vi "Process.vi"(8 "error in":errorcluster, 11 "Example Instrument UI":refnum<class "Instrument UI.Template.lvclass">) -> (0 "error out":errorcluster, 3 "Example Instrument UI out":refnum<class "Instrument UI.Template.lvclass">)   [LabVIEW 2019, in "Instrument UI.Template.lvclass"]
doc: "---------------------------------------------------------------\nJKI State Machine Objects™\nhttp://jki.net/state-machine-objects/\nCopyright (C) 2005-2015, JKI <info@jki.net>\nALL RIGHTS RESERVEDJKI State Machine Objects (SMO) 1.0.0.5\nJKI - JKI\nCopyright (c) 2016, JKI"
uses:
  Instrument UI.Template.lvclass
  C:/Program Files (x86)/National Instruments/LabVIEW 2019/vi.lib/JKI/JKI SMO/SMO/SMO.lvclass
  C:/Users/patrick/Documents/GitHub/Instrument-Framework/lvsrc/SMOs/Instrument UI/Instrument UI.lvclass
  C:/Program Files (x86)/National Instruments/LabVIEW 2019/vi.lib/JKI/JKI SMO/SMO.UI/SMO.UI.lvclass
  <vilib>/JKI/JKI SMO/SMO/Typedefs/Parent Call--Enum.ctl
  Instrument.Template/Typedefs/Instrument.Template.getAll--Cluster.ctl
  Instrument.Template/Instrument.Template.lvclass
  C:/Users/patrick/Documents/GitHub/Instrument-Framework/lvsrc/SMOs/Instrument/Instrument.lvclass
  Instrument UI.Template.UI--Cluster.ctl
  Instrument.Template/Typedefs/Instrument.Template.Configuration--Cluster.ctl
  SMOs/Configuration/Configuration.lvclass
  SMOs/Instrument UI/Instrument UI.lvclass/Instrument UI.ctl
  <vilib>/JKI/JKI SMO/SMO/SMO.lvclass/SMO.ctl
  SMOs/Instrument/Instrument.lvclass/Instrument.ctl
  614f1787-3484-4d72-b522-1f8c221dac07.vi
  064e3a37-d4cf-416d-9c97-81a00de9d50c.vi
  <vilib>/JKI/JKI SMO/SMO/Private/ReftoDVR--SMO.vi
  614f1787-3484-4d72-b522-1f8c221dac07.vi/599321bf-d042-4448-baa9-56506e4c2376.vi
  064e3a37-d4cf-416d-9c97-81a00de9d50c.vi/40046080-81aa-461f-9837-e8dd6f3bc5f2.vi
  614f1787-3484-4d72-b522-1f8c221dac07.vi/599321bf-d042-4448-baa9-56506e4c2376.vi/68c9d496-3a47-4762-a9a6-0350ec9b3b51.vi
  SMOs/Instrument/API/Send and Receive.vi
  064e3a37-d4cf-416d-9c97-81a00de9d50c.vi/40046080-81aa-461f-9837-e8dd6f3bc5f2.vi/33be0e9a-cf9b-4f8c-9dd9-f20244ed4396.vi
  614f1787-3484-4d72-b522-1f8c221dac07.vi/599321bf-d042-4448-baa9-56506e4c2376.vi/68c9d496-3a47-4762-a9a6-0350ec9b3b51.vi/238fe6a9-6a91-4c49-8d30-1c3fb86c5f8a.vi
  614f1787-3484-4d72-b522-1f8c221dac07.vi/599321bf-d042-4448-baa9-56506e4c2376.vi/68c9d496-3a47-4762-a9a6-0350ec9b3b51.vi/b5f16ff4-5c24-4e80-bad9-cd4679a5a0b8.vi
  064e3a37-d4cf-416d-9c97-81a00de9d50c.vi/40046080-81aa-461f-9837-e8dd6f3bc5f2.vi/33be0e9a-cf9b-4f8c-9dd9-f20244ed4396.vi/94746ab4-2c68-4577-8c39-bf3a51064162.vi
  064e3a37-d4cf-416d-9c97-81a00de9d50c.vi/40046080-81aa-461f-9837-e8dd6f3bc5f2.vi/33be0e9a-cf9b-4f8c-9dd9-f20244ed4396.vi/78597d36-8981-4427-a4ab-fc029080c8ad.vi
  SMOs/Instrument/API/Enum to String.vi
  SMOs/RemoteControl/API/Send and Receive.vi
  <vilib>/Utility/Data Type/Get Type Information.vi
  <vilib>/JDP Science/JSONtext/JSON text to Variant.vi
  SMOs/Instrument/Instrument.lvclass
  <vilib>/JDP Science/JSONtext/LVClass Serializer/JSONtext LVClass Serializer.lvclass
  SMOs/Instrument UI/Instrument UI.lvclass
  <vilib>/JKI/JKI SMO/SMO/SMO.lvclass
  <vilib>/JKI/JKI SMO/SMO.UI/SMO.UI.lvclass
panel:
  in  "Parameter 2":string
  out "Numeric":u32
  in  "Set Parameter":bool
  in  "Parameter":dbl
  in  "STOP":bool
  out "SMO string":string
  out "SMO Boolean":bool
  out "Logger SMO":dbl
  out "Levy 1":dbl
  # "#todo\nmake UI here. maybe include a nice picture of the hardware?"
  # "#todo\nadd buttons to do stuff (e.g., change a setting)\nButtons should trigger an event"
  # "#todo\nresize this box if you want your UI to be different size"
  # "SMO UI Template"
  # "For instructions on how to use the JKI State Machine Objects, examples and video tutorials, visit:\nhttp://jki.net/state-machine-objects/\n\nJKI State Machine Objects™\nhttp://jki.net/state-machine-objects/\nCopyright (C) 2005-2015, JKI <info@jki.net>\nALL RIGHTS RESERVED"
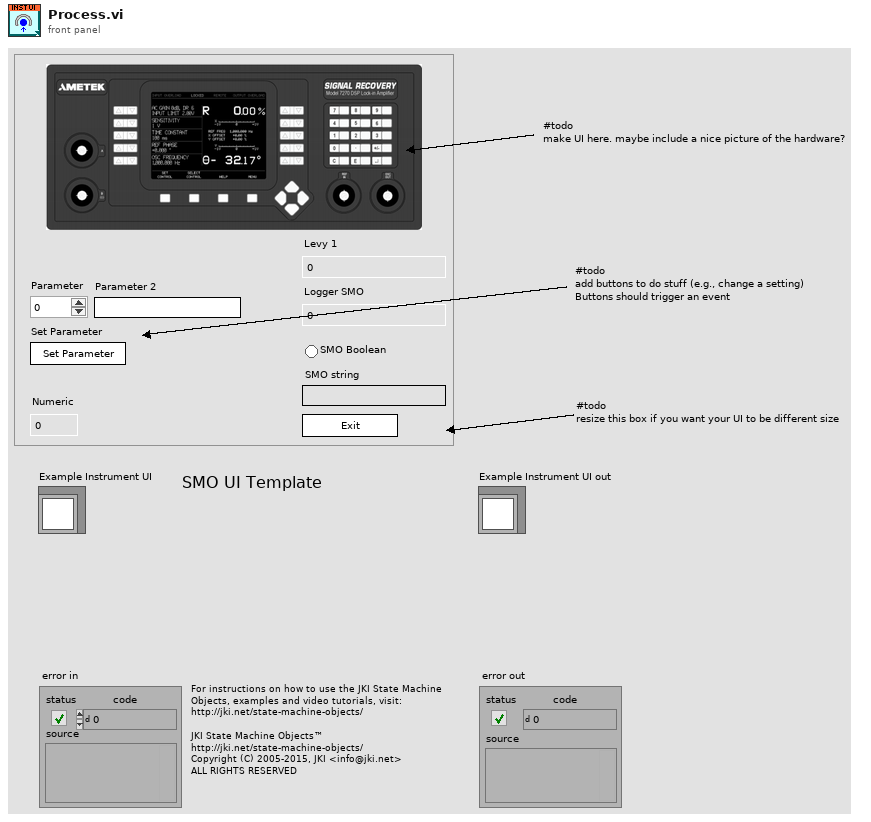
[diagram p1: front panel]
types:
  T1 = typedef "SMO.lvclass/Parent Call--Enum.ctl" = enum16{"Allows parent to run", "Does not request parent to run"}
  T2 = enum32{"invalid app kind", "Development System", "Run Time System", "Student Edition", "Embedded LabVIEW", "Evaluation", "Custom"}
  T3 = enum32{"Invalid", "Standard", "Closed", "Hidden", "Minimized", "Maximized"}
  T4 = typedef "Instrument.Template.lvclass/Instrument.Template.Configuration--Cluster.ctl" = cluster{"Example Setting 1":dbl, "Example Setting 2":dbl, "Example Setting 3":string}
  T5 = typedef "Instrument.Template.lvclass/Instrument.Template.getAll--Cluster.ctl" = cluster{"Levy 1":dbl, "Logger SMO":dbl, "SMO Boolean":bool, "SMO String":string}
  T6 = typedef "Instrument UI.Template.lvclass/Instrument UI.Template.UI--Cluster.ctl" = cluster{"Parameter":dbl, "Parameter 2":string}
  T7 = cluster{"Core":cluster{"Current VI Reference":refnum<vi>, "Close Panel on Exit?":bool, "error":errorcluster}, "Instrument UI":refnum<class "Instrument UI.Template.lvclass">, "Instrument":refnum<class "Instrument.Template.lvclass">, "Configuration":refnum<class "Configuration.lvclass">, "Config Cluster":T4, "getAll":T5, "UI Cluster":T6}
  T8 = cluster{"Current VI Reference":refnum<vi>, "Close Panel on Exit?":bool, "error":errorcluster}
  T9 = typedef "SMO.lvclass/Protected Events.ctl" = cluster{"StopProcesses":refnum<user-event>, "AbortProcesses":refnum<user-event>, "Config Changed":refnum<user-event>, "Dependency":refnum<user-event>}
  T10 = typedef "Instrument.lvclass/PublicEvents--Cluster.ctl" = cluster{"MessageFromProcess":refnum<user-event>}
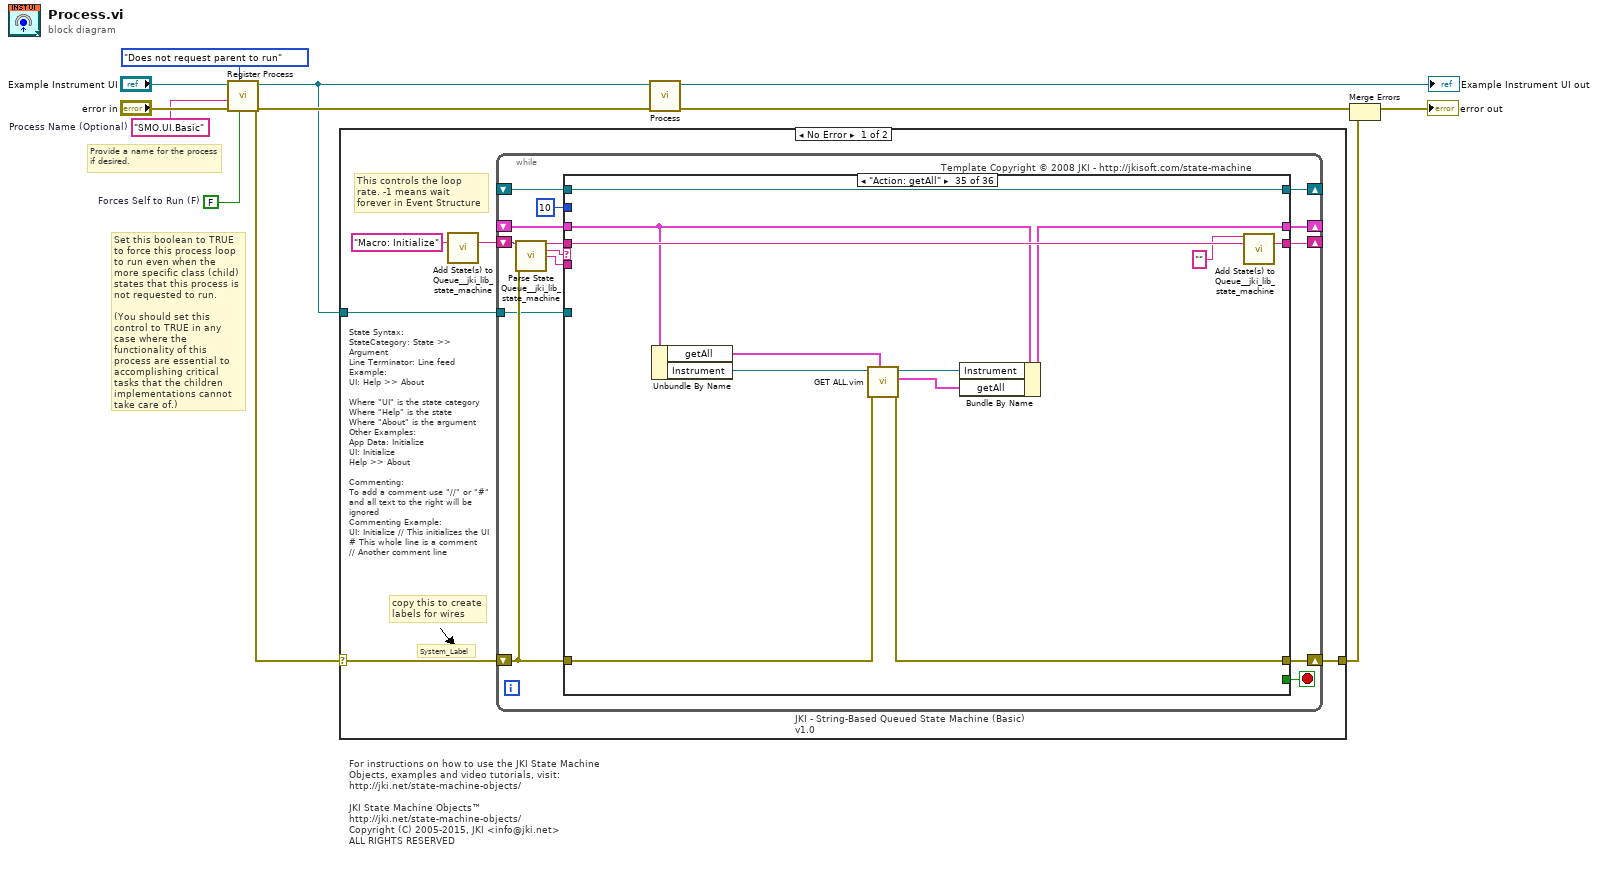
[diagram p0: block diagram]
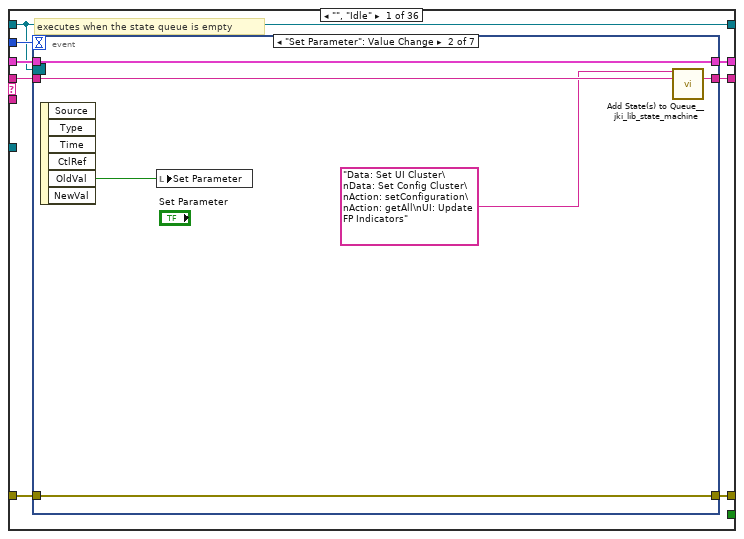
[diagram p2: hidden frame]
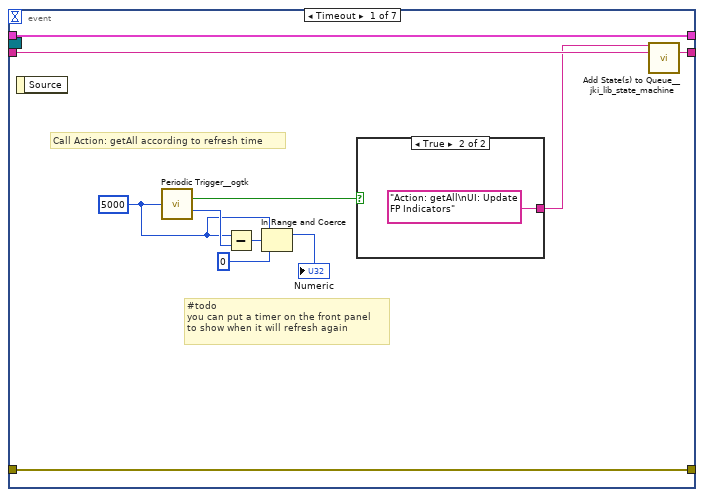
[diagram p3: hidden frame]
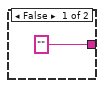
[diagram p4: hidden frame]
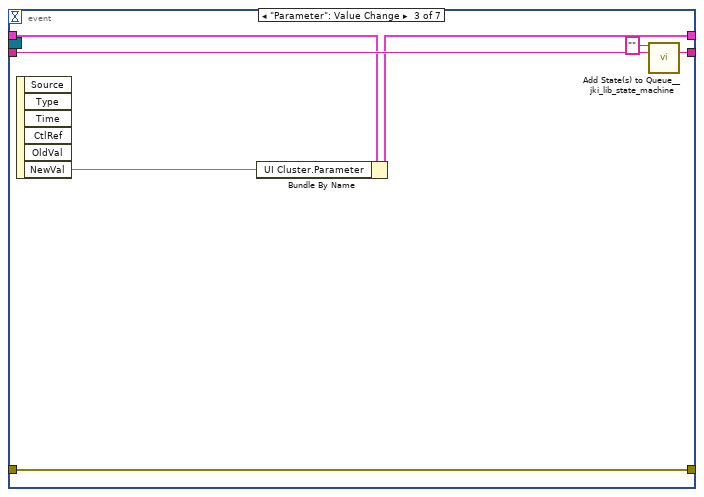
[diagram p5: hidden frame]
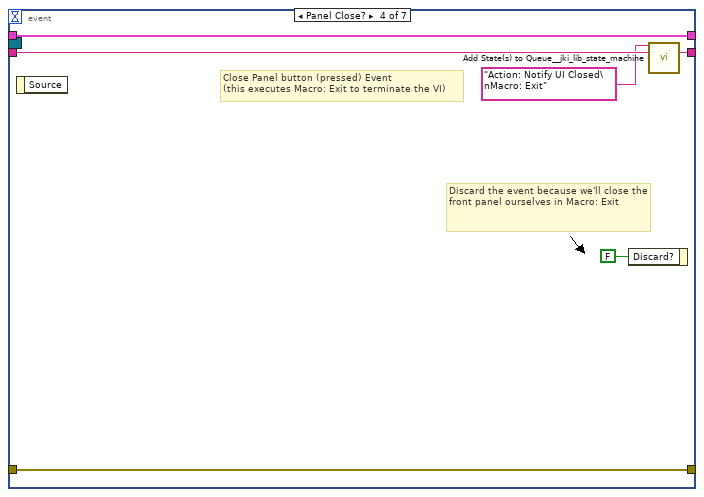
[diagram p6: hidden frame]
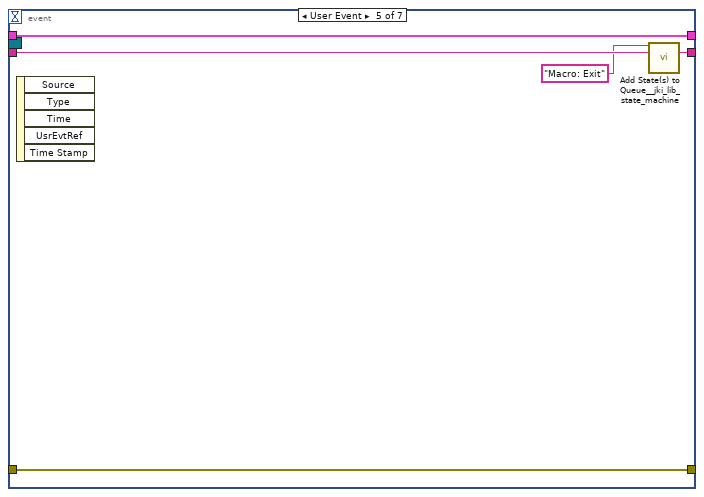
[diagram p7: hidden frame]
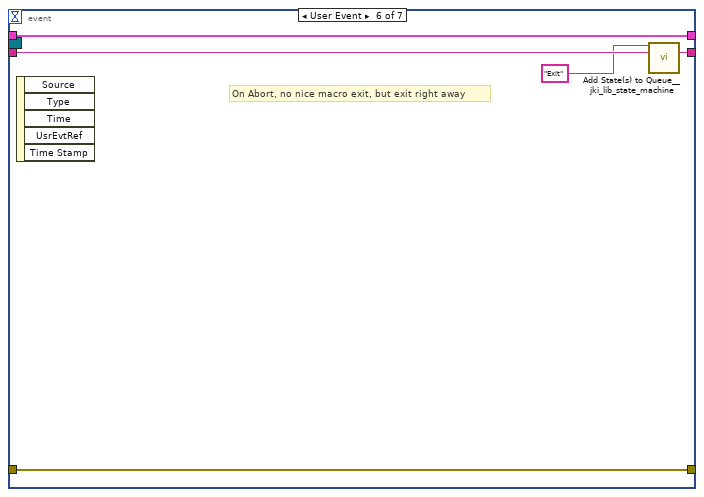
[diagram p8: hidden frame]
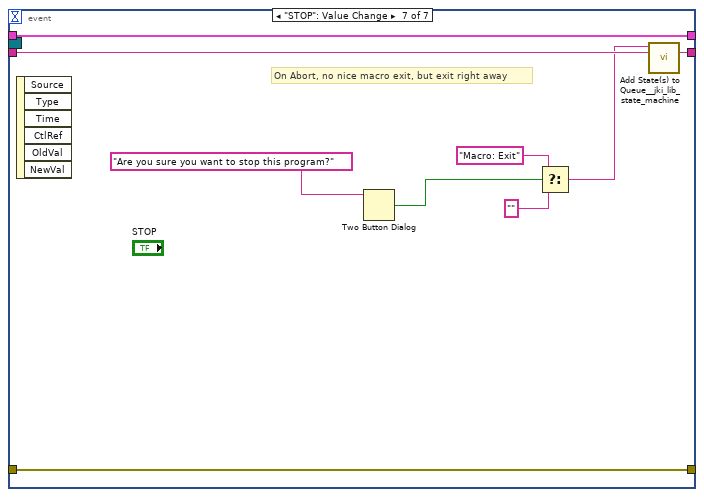
[diagram p9: hidden frame]
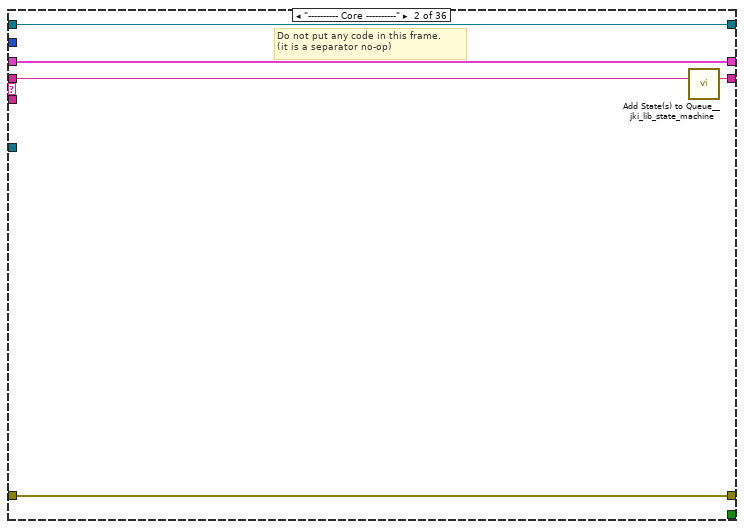
[diagram p10: hidden frame]
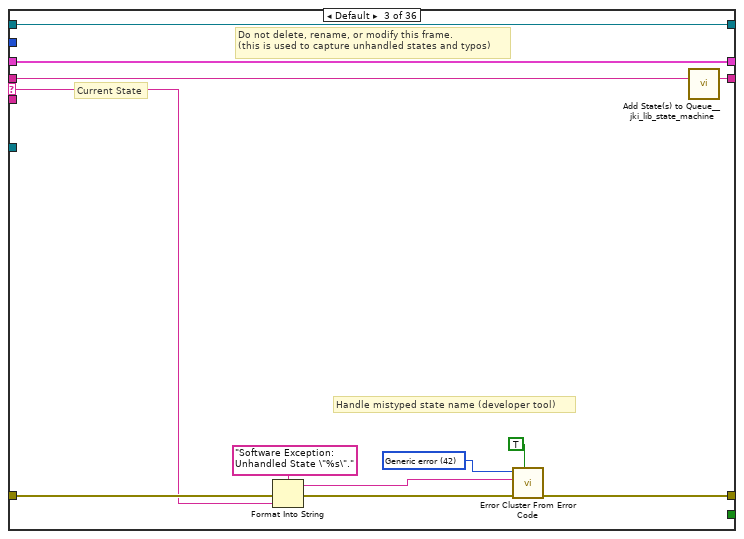
[diagram p11: hidden frame]
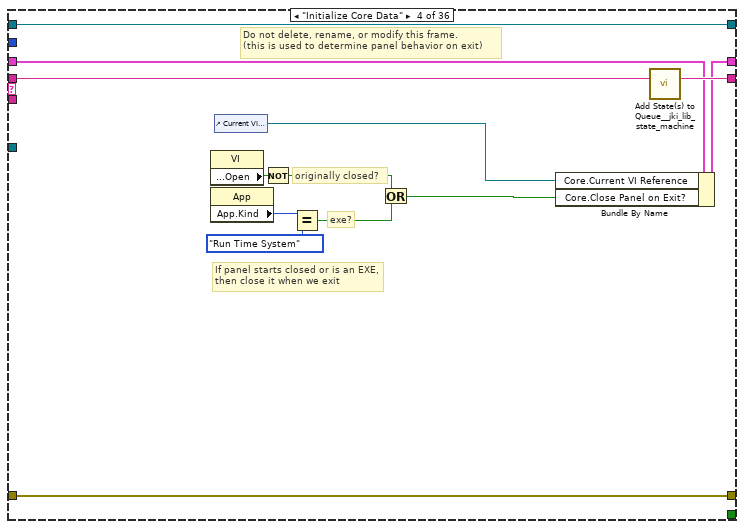
[diagram p12: hidden frame]
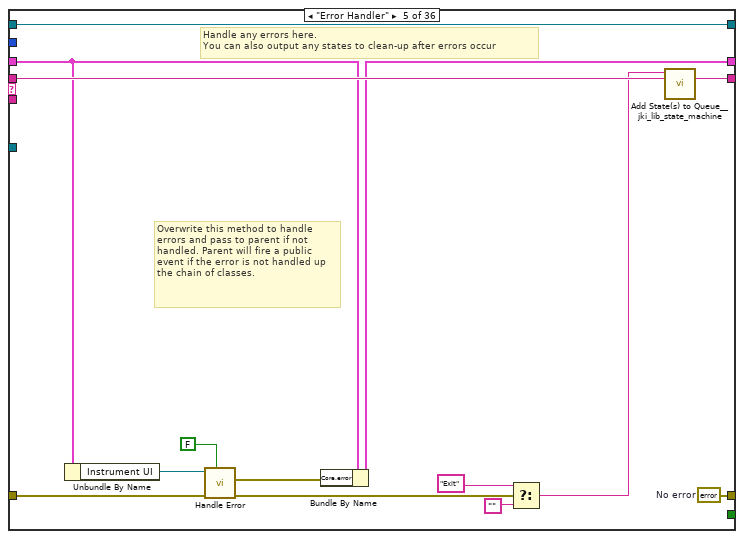
[diagram p13: hidden frame]
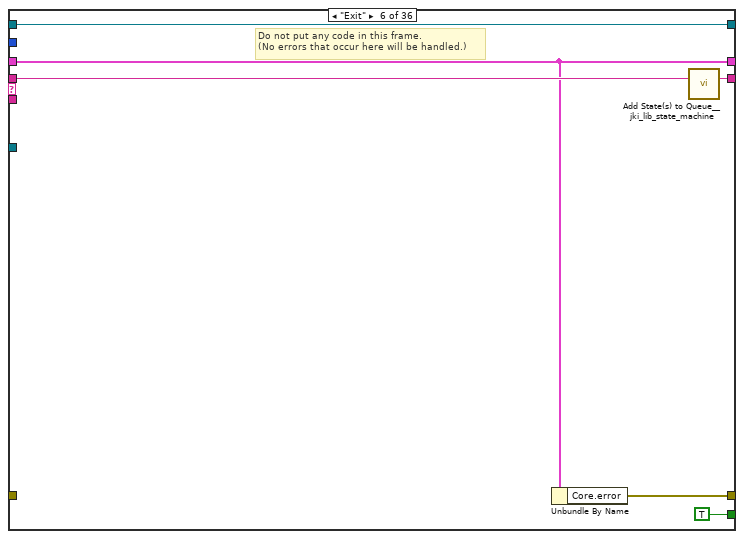
[diagram p14: hidden frame]
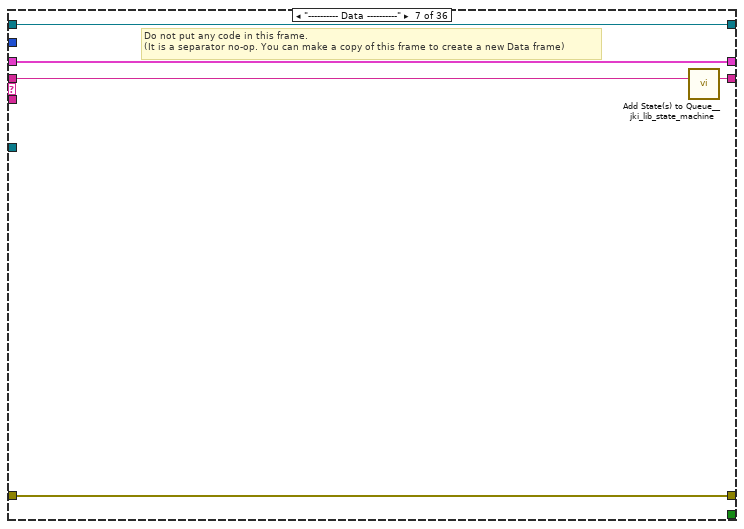
[diagram p15: hidden frame]
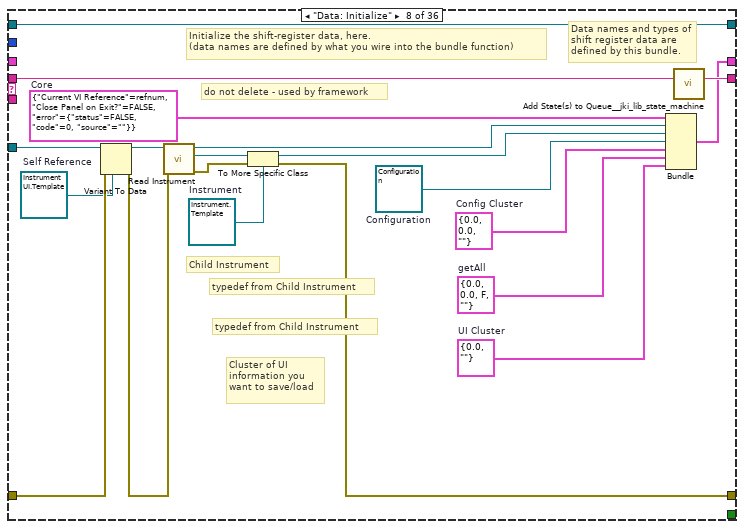
[diagram p16: hidden frame]
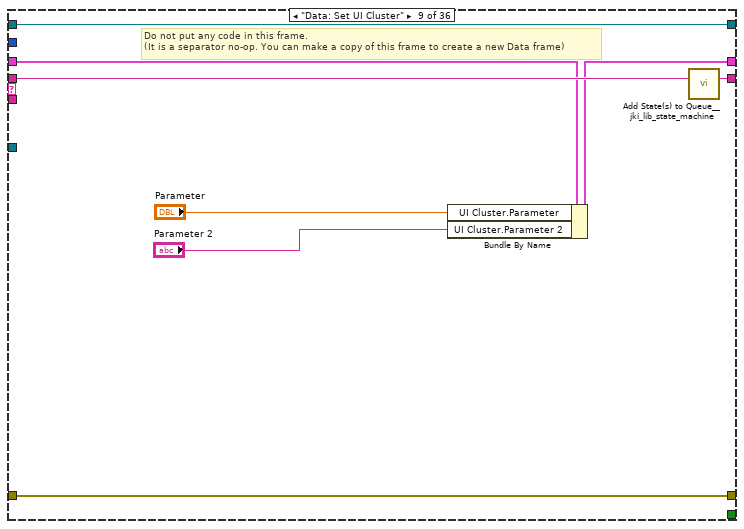
[diagram p17: hidden frame]
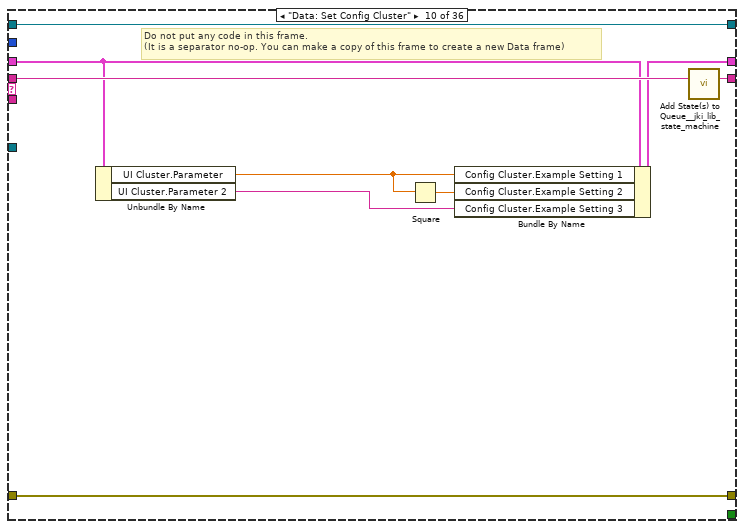
[diagram p18: hidden frame]
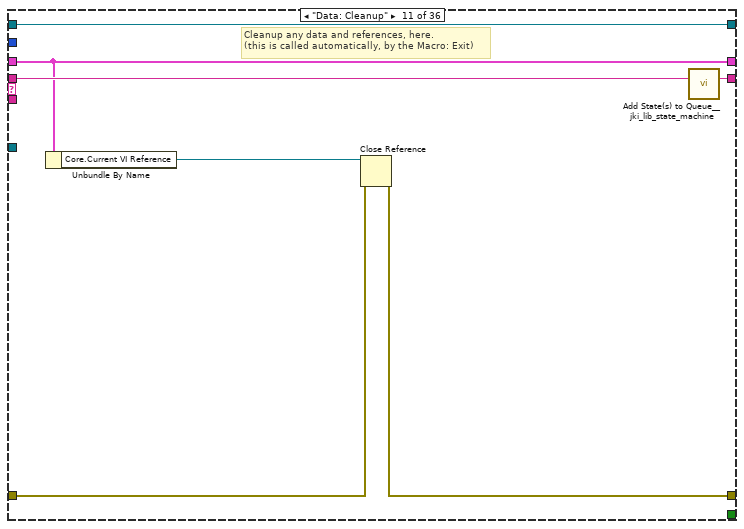
[diagram p19: hidden frame]
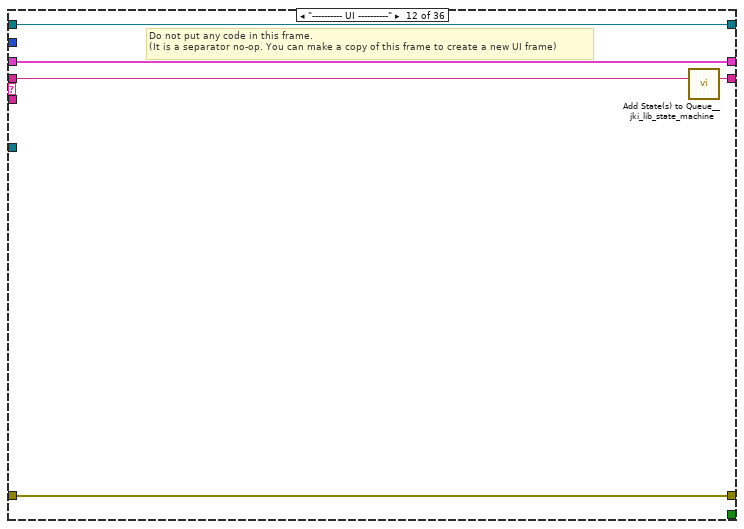
[diagram p20: hidden frame]
diagram:
  w2 = FALSE  # Forces Self to Run (F)
  w1 = "SMO.UI.Basic"  # Process Name (Optional)
  # "Provide a name for the process\nif desired."
  # "Set this boolean to TRUE to force this process loop to run even when the more specific class (child) states that this process is not requested to run.\n\n(You should set this control to TRUE in any case where the functionality of this process are essential to accomplishing critical tasks that the children implementations cannot take care of.)"
  # "For instructions on how to use the JKI State Machine Objects, examples and video tutorials, visit:\nhttp://jki.net/state-machine-objects/\n\nJKI State Machine Objects™\nhttp://jki.net/state-machine-objects/\nCopyright (C) 2005-2015, JKI <info@jki.net>\nALL RIGHTS RESERVED"
  n1 = call <vilib>:"Register Process.vi"("Forces Self to Run (F)"=w2, "Parent Call"=Parent_Call--Enum."Does not request parent to run", "error in (no error)"="error in", "Process Name (optional)"=w1, "SMO"="Example Instrument UI") -> ("error out"=w8:errorcluster, "SMO out"=w7:refnum<class "Instrument UI.Template.lvclass">)  [unwired: 5 in]
  n2 = case shown="No Error" w8 {
    selector: w8 -> [w13 w430]
    tunnel: w7 -> [w14 _]
    tunnel: [w12 w430] -> w4
    frame No Error {
      # "State Syntax:\nStateCategory: State >> Argument\nLine Terminator: Line feed\nExample:\nUI: Help >> About\n\nWhere \"UI\" is the state category\nWhere \"Help\" is the state\nWhere \"About\" is the argument\nOther Examples:\nApp Data: Initialize\nUI: Initialize\nHelp >> About\n\nCommenting:\nTo add a comment use \"//\" or \"#\" and all text to the right will be ignored\nCommenting Example:\nUI: Initialize // This initializes the UI\n# This whole line is a comment\n// Another comment line"
      # "copy this to create labels for wires"
      # "This controls the loop rate. -1 means wait forever in Event Structure"
      # "System_Label"
      n3 = call <vilib>:"Add State(s) to Queue__jki_lib_state_machine.vi"("State(s) in (\"\")"="Macro: Initialize") -> ("States Out"=w16:string)  [unwired: 14 in]
      n4 = while "JKI - String-Based Queued State Machine (Basic) v1.0" {
        shift-right: [w23] -> _
        shift-left: _ -> [w22]
        shift-right: [w26] -> w12
        shift-left: w13 -> [w20]
        shift-right: [w25] -> _
        shift-left: w16 -> [w27]
        tunnel: w14 -> [w19]
        shift-right: [w18] -> _
        shift-left: _ -> [w17]
        stop <- w24 stop-if-true
        # "Template Copyright © 2008 JKI - http://jkisoft.com/state-machine"
        n5 = call <vilib>:"Parse State Queue__jki_lib_state_machine.vi"("State Queue"=w27, "Error In (no error)"=w20) -> ("Remaining States"=w29:string, "Current State"=w30:string, "Arguments"=w28:string)  [unwired: 11 in]
        n6 = case shown="\"Action: getAll\"" w30 {
          selector: w30 -> [_ _ w96 _ _ _ _ _ _ _ _ _ _ _ _ _ _ _ _ _ _ _ _ _ _ _ _ _ _ _ _ _ _ _ _ _]
          tunnel: w29 -> [w38 w94 w100 w119 w133 w139 w144 w164 w172 w181 w188 w193 w200 w207 w217 w224 w240 w272 w281 w287 w293 w308 w313 w324 w331 w336 w349 w355 w360 w372 w380 w392 w399 w406 w418 w429]
          tunnel: w28 -> [_ _ _ _ _ _ _ _ _ _ _ _ _ _ _ w218 w234 _ _ _ _ _ _ _ _ _ _ _ _ _ _ _ _ _ _ _]
          tunnel: w22 -> [w36 w91 w98 w110 w122 w135 w141 _ w168 w177 w182 w190 w198 w203 w208 w222 w236 w269 w277 w284 w290 w295 w310 w321 w326 w333 w347 w353 w357 w363 w377 w383 w395 w400 w410 w421]
          tunnel: [w35 w92 w102 w116 w124 w134 w142 w146 w170 w179 w184 w191 w195 w205 w209 w219 w237 w270 w279 w285 w291 w306 w311 w315 w327 w334 w342 w350 w358 w367 w375 w384 w396 w401 w415 w426] -> w26
          tunnel: w20 -> [w34 w92 w101 w116 w129 _ w142 w161 w170 w179 w185 w191 w196 w205 w209 w220 w238 w270 w279 w285 w291 w306 w311 w316 w328 w334 w344 w351 w358 w365 w373 w385 w396 w402 w411 w422]
          tunnel: [w37 w93 w99 w118 w132 w138 w143 w163 w171 w180 w187 w192 w199 w206 w216 w223 w239 w271 w280 w286 w292 w307 w312 w323 w330 w335 w348 w354 w359 w371 w379 w391 w398 w405 w417 w428] -> w25
          tunnel: [_ _ _ _ _ TRUE _ _ _ _ _ _ _ _ _ _ _ _ _ _ _ _ _ _ _ _ _ _ _ _ _ _ _ _ _ _] -> w24
          tunnel: [w33 w91 w98 w117 w121 w135 w141 w162 w167 w176 w182 w190 w198 w203 w208 w222 w236 w269 w277 w284 w290 w295 w310 w321 w326 w333 w347 w353 w357 w369 w377 w381 w394 w400 w412 w423] -> w23
          tunnel: 10 ("Timeout") -> [w32 _ _ _ _ _ _ _ _ _ _ _ _ _ _ _ _ _ _ _ _ _ _ _ _ _ _ _ _ _ _ _ _ _ _ _]
          tunnel: w19 -> [_ _ _ _ _ _ _ w159 _ _ _ _ _ _ _ _ _ _ _ _ _ _ _ _ _ _ _ _ _ _ _ _ _ _ _ _]
          tunnel: [w31 w90 w95 w107 w131 w136 w140 w158 w169 w178 w183 w189 w197 w204 w215 w221 w233 w268 w278 w283 w289 w300 w309 w322 w329 w332 w346 w352 w356 w370 w378 w390 w397 w404 w416 w427] -> w18
          tunnel: w17 -> [w31 w90 w95 w107 w131 w136 w140 w158 w169 w178 w183 w189 w197 w204 w215 w221 w233 w268 w278 w283 w289 w300 w309 w322 w329 w332 _ w352 w356 w370 w378 w390 w397 w404 w416 w427]
          frame "", "Idle" {
            # "executes when the state queue is empty"
            n7 = event shown="[1] \"Set Parameter\": Value Change" {
              selector: w31 -> [_ _ _ _ _ _ _]
              dyn-events: _ -> [_ _ _ _ _ _ _]
              timeout: w32 -> [_ _ _ _ _ _ _]
              tunnel: w38 -> [w49 w57 w64 w70 w75 w80 w89]
              tunnel: [w48 w56 w63 w69 w74 w79 w88] -> w37
              tunnel: w36 -> [w46 w54 w60 w66 w72 w77 w86]
              tunnel: [w47 w55 w62 w65 w73 w78 w87] -> w35
              tunnel: w34 -> [w47 w55 w62 w65 w73 w78 w87]
              tunnel: [w46 w54 w59 w66 w72 w77 w86] -> w33
              event Timeout {
                w40 = u32 5000 ("time (ms)")
                # "#todo\nyou can put a timer on the front panel\nto show when it will refresh again"
                # "Call Action: getAll according to refresh time"
                n8 = event-data() -> ()  [unwired: 1 in, 1 out]
                n9 = call <userlib>:"Periodic Trigger__ogtk.vi"("time (ms)"=w40) -> ("Triggered"=w44:bool, "timer value"=w43:u32)  [unwired: 12 in, 1 out]
                n10 = Subtract(x=w40, y=w43) -> (x-y=w42:u32)
                n11 = In Range and Coerce(upper limit=w40, x=w42, lower limit=u32 0) -> (coerced(x)=→"Numeric":u32)  [unwired: 1 out]
                n12 = case shown="True" w44 {
                  tunnel: ["" ("State(s) in Front (\"\")") "Action: getAll\nUI: Update FP Indicators" ("State(s) in Front (\"\")")] -> w45
                  frame False {
                  }
                  frame True {
                  }
                }
                n13 = call <vilib>:"Add State(s) to Queue__jki_lib_state_machine.vi"("State(s) in Front (\"\")"=w45, "State(s) in (\"\")"=w49) -> ("States Out"=w48:string)  [unwired: 13 in]
              }
              event "Set Parameter": Value Change {
                n14 = event-data() -> ("OldVal"=w53:bool)  [unwired: 1 in, 5 out]
                n15 = local write "Set Parameter"(w53) -> ()
                n16 = call <vilib>:"Add State(s) to Queue__jki_lib_state_machine.vi"("State(s) in Front (\"\")"="Data: Set UI Cluster\nData: Set Config Cluster\nAction: setConfiguration\nAction: getAll\nUI: Update FP Indicators" ("State(s) in Front (\"\")"), "State(s) in (\"\")"=w57) -> ("States Out"=w56:string)  [unwired: 13 in]
              }
              event "Parameter": Value Change {
                n17 = event-data() -> ("NewVal"=w61:dbl)  [unwired: 1 in, 5 out]
                n18 = Bundle By Name(cluster=w60, "UI Cluster.Parameter"=w61) -> (w59:T7)
                n19 = call <vilib>:"Add State(s) to Queue__jki_lib_state_machine.vi"("State(s) in Front (\"\")"="" ("State(s) in Front (\"\")"), "State(s) in (\"\")"=w64) -> ("States Out"=w63:string)  [unwired: 13 in]
              }
              event Panel Close? {
                # "Discard the event because we'll close the front panel ourselves in Macro: Exit"
                # "Close Panel button (pressed) Event\n(this executes Macro: Exit to terminate the VI)"
                n20 = event-data() -> ()  [unwired: 1 in, 1 out]
                n21 = event-data("Discard?"=FALSE) -> ()  [unwired: 1 in, 1 out]
                n22 = call <vilib>:"Add State(s) to Queue__jki_lib_state_machine.vi"("State(s) in Front (\"\")"="Action: Notify UI Closed\nMacro: Exit", "State(s) in (\"\")"=w70) -> ("States Out"=w69:string)  [unwired: 13 in]
              }
              event User Event {
                n23 = event-data() -> ()  [unwired: 1 in, 5 out]
                n24 = call <vilib>:"Add State(s) to Queue__jki_lib_state_machine.vi"("State(s) in Front (\"\")"="Macro: Exit", "State(s) in (\"\")"=w75) -> ("States Out"=w74:string)  [unwired: 13 in]
              }
              event User Event {
                # "On Abort, no nice macro exit, but exit right away"
                n25 = event-data() -> ()  [unwired: 1 in, 5 out]
                n26 = call <vilib>:"Add State(s) to Queue__jki_lib_state_machine.vi"("State(s) in Front (\"\")"="Exit", "State(s) in (\"\")"=w80) -> ("States Out"=w79:string)  [unwired: 13 in]
              }
              event "STOP": Value Change {
                # "On Abort, no nice macro exit, but exit right away"
                n27 = event-data() -> ()  [unwired: 1 in, 6 out]
                n28 = Two Button Dialog(message="Are you sure you want to stop this program?") -> (T button?=w85:bool)  [unwired: 2 in]
                n29 = Select(t="Macro: Exit", s=w85, f="") -> (s? t:f=w81:string)
                n30 = call <vilib>:"Add State(s) to Queue__jki_lib_state_machine.vi"("State(s) in Front (\"\")"=w81, "State(s) in (\"\")"=w89) -> ("States Out"=w88:string)  [unwired: 13 in]
              }
            }
          }
          frame "---------- Core ----------" {
            # "Do not put any code in this frame.\n(it is a separator no-op)"
            n31 = call <vilib>:"Add State(s) to Queue__jki_lib_state_machine.vi"("State(s) in (\"\")"=w94) -> ("States Out"=w93:string)  [unwired: 14 in]
          }
          frame Default {
            w105 = 42 items=["No error", "Argument error", "Memory is full", "Out of zone", "End of file", "File already open", "Generic file I/O error", "File not found", "File permission error", "Disk is full", "Duplicate path", "Too many files open", "System feature not enabled", "Resource file not found", "Cannot add resource", "Resource not found", "Image not found", "Image memory error", "Pen does not exist", "Config type invalid", "Config token not found", "Config parse error", "Config memory error", "Bad external code format", "Bad external code offset", "External code not present", "Null window", "Destroy window error", "Null menu", "Print aborted", "Bad print record", "Print driver error", "Windows error during printing", "Memory error during printing", "Print dialog error", "Generic print error", "Invalid device refnum", "Device not found", "Device parameter error", "Device unit error", "Cannot open device", "Device call aborted", "Generic error", "Cancelled by user", "Object ID too low", "Object ID too high", "Object not in heap", "Unknown heap", "Unknown object (invalid DefProc)", "Unknown object (DefProc not in table)", "Message out of range", "Invalid (null) method", "Unknown message", "Manager call not supported", "Bad address", "Network operation in progress", "Network operation timed out", "Connection is busy", "Network attribute not supported", "Network error", "Address in use", "System out of memory", "Connection aborted", "Connection refused", "Not connected", "Already connected", "Connection closed", "Initialization error (interapplication manager)", "Bad occurrence", "Wait on unbound occurrence handler", "Occurrence queue overflow", "Datalog type conflict", "Unused", "Unrecognized type (interapplication manager)", "Memory corrupt", "Failed to make temporary DLL", "Old CIN version", "Drag socket not found", "Failed to load drop-object", "Failed to register OLE object", "Failed to release OLE object", "Format specifier type mismatch", "Unknown format specifier", "Too few format specifiers", "Too many format specifiers", "Scan failed", "Newer CIN version", "Error converting to variant", "Runtime menu error", "Password tampered", "Variant attribute not found", "Incompatible variant data type", "Event data is not available", "Event Store is not present", "Occurrence is not found", "Event Queue is not created", "Event info is not available", "Refnum passed is NULL", "Error retrieving Class GUID", "Error retrieving CoClass GUID", "Error retrieving TypeLib GUID.", "Bad built application magic bytes.", "Specific driver is different from the specific driver associated with the Logical Name.", "There is no session opened to the class driver.", "Max Error", "MAX - Error with config objects", "MAX - Error loading configuration", "MAX - Group not supported"]
            # "Current State"
            # "Do not delete, rename, or modify this frame.\n(this is used to capture unhandled states and typos)"
            # "Handle mistyped state name (developer tool)"
            n32 = Format Into String(format string="Software Exception: Unhandled State \"%s\"." ("message"), error in=w101, w96) -> (resulting string=w104:string, error out=w103:errorcluster)  [unwired: 1 in]
            n33 = call <vilib>:"Error Cluster From Error Code.vi"("show call chain? (False)"=TRUE, "error in (no error)"=w103, "error message (\"\")"=w104, "error code (0)"=w105) -> ("error out"=w102:errorcluster)  [unwired: 5 in]
            n34 = call <vilib>:"Add State(s) to Queue__jki_lib_state_machine.vi"("State(s) in (\"\")"=w100) -> ("States Out"=w99:string)  [unwired: 14 in]
          }
          frame "Initialize Core Data" {
            # "Do not delete, rename, or modify this frame.\n(this is used to determine panel behavior on exit)"
            # "originally closed?"
            # "exe?"
            # "If panel starts closed or is an EXE, then close it when we exit"
            n35 = property class="VI"() -> ("Front Panel.Open"=w115:bool)  [unwired: 2 in, 2 out]
            n36 = property class="App"() -> ("App.Kind"=w114:T2)  [unwired: 2 in, 2 out]
            n37 = control-ref of="Current VI Reference"() -> (w108:refnum<vi>)
            n38 = Not(x=w115) -> (.not. x?=w112:bool)
            n39 = Equal?(x=w114, y=T2."Run Time System" ("Application:Kind")) -> (x = y?=w111:bool)
            n40 = Or(x=w112, y=w111) -> (x .or. y?=w109:bool)
            n41 = Bundle By Name(cluster=w110, "Core.Current VI Reference"=w108, "Core.Close Panel on Exit?"=w109) -> (w117:T7)
            n42 = call <vilib>:"Add State(s) to Queue__jki_lib_state_machine.vi"("State(s) in (\"\")"=w119) -> ("States Out"=w118:string)  [unwired: 14 in]
          }
          frame "Error Handler" {
            w124 = errorcluster {"status"=FALSE, "code"=0, "source"=""}  # No error
            # "Overwrite this method to handle errors and pass to parent if not handled. Parent will fire a public event if the error is not handled up the chain of classes."
            # "Handle any errors here.\nYou can also output any states to clean-up after errors occur"
            n43 = Unbundle By Name(w122) -> ("Instrument UI"=w130:refnum<class "Instrument UI.Template.lvclass">)
            n44 = call-dynamic "Handle Error.vi"("Stop on Unhandled Error (T)"=FALSE, "error in"=w129, "SMO"=w130) -> ("handling error"=w125:errorcluster, "Unhandled error"=w123:errorcluster)  [unwired: 6 in, 1 out]
            n45 = Bundle By Name(cluster=w122, "Core.error"=w123) -> (w121:T7)
            n46 = Select(t="Exit", s=w125, f="") -> (s? t:f=w126:string)
            n47 = call <vilib>:"Add State(s) to Queue__jki_lib_state_machine.vi"("State(s) in Front (\"\")"=w126, "State(s) in (\"\")"=w133) -> ("States Out"=w132:string)  [unwired: 13 in]
          }
          frame "Exit" {
            # "Do not put any code in this frame.\n(No errors that occur here will be handled.)"
            n48 = Unbundle By Name(w135) -> ("Core.error"=w134:errorcluster)
            n49 = call <vilib>:"Add State(s) to Queue__jki_lib_state_machine.vi"("State(s) in (\"\")"=w139) -> ("States Out"=w138:string)  [unwired: 14 in]
          }
          frame "---------- Data ----------" {
            # "Do not put any code in this frame.\n(It is a separator no-op. You can make a copy of this frame to create a new Data frame)"
            n50 = call <vilib>:"Add State(s) to Queue__jki_lib_state_machine.vi"("State(s) in (\"\")"=w144) -> ("States Out"=w143:string)  [unwired: 14 in]
          }
          frame "Data: Initialize" {
            w145 = refnum<class "Configuration.lvclass"> refnum  # Configuration
            w148 = T4 {"Example Setting 1"=0.0, "Example Setting 2"=0.0, "Example Setting 3"=""}  # Config Cluster
            w150 = T6 {"Parameter"=0.0, "Parameter 2"=""}  # UI Cluster
            w152 = refnum<class "Instrument.Template.lvclass"> refnum  # Instrument
            w156 = T5 {"Levy 1"=0.0, "Logger SMO"=0.0, "SMO Boolean"=FALSE, "SMO String"=""}  # getAll
            w157 = T8 {"Current VI Reference"=refnum, "Close Panel on Exit?"=FALSE, "error"={"status"=FALSE, "code"=0, "source"=""}}  # Core
            w160 = refnum<class "Instrument UI.Template.lvclass"> refnum  # Self Reference
            # "typedef from Child Instrument"
            # "Cluster of UI\ninformation you\nwant to save/load"
            # "Child Instrument"
            # "typedef from Child Instrument"
            # "do not delete - used by framework"
            # "Data names and types of shift register data are defined by this bundle."
            # "Initialize the shift-register data, here.\n(data names are defined by what you wire into the bundle function)"
            n51 = Variant To Data(error in=w161, type=w160, Variant=w159) -> (data=w154:refnum<class "Instrument UI.Template.lvclass">, error out=w155:errorcluster)
            n52 = call "Read Instrument.vi"("error in (no error)"=w155, "Instrument UI in"=w154) -> ("error out"=w149:errorcluster, "Instrument"=w151:refnum<class "Instrument.lvclass">, "Instrument UI"=w153:refnum<class "Instrument UI.Template.lvclass">)  [unwired: 7 in]
            n53 = To More Specific Class(target class=w152, reference=w151, error in=w149) -> (specific class reference=w147:refnum<class "Instrument.Template.lvclass">, error out=w146:errorcluster)
            n54 = Bundle("Core"=w157, "Instrument UI"=w153, "Instrument"=w147, "Configuration"=w145, "Config Cluster"=w148, "getAll"=w156, "UI Cluster"=w150) -> (w162:T7)  [unwired: 1 in]
            n55 = call <vilib>:"Add State(s) to Queue__jki_lib_state_machine.vi"("State(s) in (\"\")"=w164) -> ("States Out"=w163:string)  [unwired: 14 in]
          }
          frame "Data: Set UI Cluster" {
            # "Do not put any code in this frame.\n(It is a separator no-op. You can make a copy of this frame to create a new Data frame)"
            n56 = Bundle By Name(cluster=w168, "UI Cluster.Parameter"="Parameter", "UI Cluster.Parameter 2"="Parameter 2") -> (w167:T7)
            n57 = call <vilib>:"Add State(s) to Queue__jki_lib_state_machine.vi"("State(s) in (\"\")"=w172) -> ("States Out"=w171:string)  [unwired: 14 in]
          }
          frame "Data: Set Config Cluster" {
            # "Do not put any code in this frame.\n(It is a separator no-op. You can make a copy of this frame to create a new Data frame)"
            n58 = Unbundle By Name(w177) -> ("UI Cluster.Parameter"=w174:dbl, "UI Cluster.Parameter 2"=w175:string)
            n59 = Square(x=w174) -> (x^2=w173:dbl)
            n60 = Bundle By Name(cluster=w177, "Config Cluster.Example Setting 1"=w174, "Config Cluster.Example Setting 2"=w173, "Config Cluster.Example Setting 3"=w175) -> (w176:T7)
            n61 = call <vilib>:"Add State(s) to Queue__jki_lib_state_machine.vi"("State(s) in (\"\")"=w181) -> ("States Out"=w180:string)  [unwired: 14 in]
          }
          frame "Data: Cleanup" {
            # "Cleanup any data and references, here.\n(this is called automatically, by the Macro: Exit)"
            n62 = Unbundle By Name(w182) -> ("Core.Current VI Reference"=w186:refnum<vi>)
            n63 = Close Reference(reference=w186, error in (no error)=w185) -> (error out=w184:errorcluster)
            n64 = call <vilib>:"Add State(s) to Queue__jki_lib_state_machine.vi"("State(s) in (\"\")"=w188) -> ("States Out"=w187:string)  [unwired: 14 in]
          }
          frame "---------- UI ----------" {
            # "Do not put any code in this frame.\n(It is a separator no-op. You can make a copy of this frame to create a new UI frame)"
            n65 = call <vilib>:"Add State(s) to Queue__jki_lib_state_machine.vi"("State(s) in (\"\")"=w193) -> ("States Out"=w192:string)  [unwired: 14 in]
          }
          frame "UI: Initialize" {
            # "size window to decoration box on front panel"
            # "Initialize the User Interface, here.\n(this is called automatically, by the Macro: Init)"
            n66 = invoke on="STOP" class="Bool (strict)" method="Reinit To Default"() -> ()  [unwired: 3 in, 3 out]
            n67 = call <userlib>:"Fit VI window to Largest Dec__ogtk.vi"("error in (no error)"=w196, "border spacing (2 px)"=0) -> ("error out"=w195:errorcluster)  [unwired: 4 in, 1 out]
            n68 = call <vilib>:"Add State(s) to Queue__jki_lib_state_machine.vi"("State(s) in (\"\")"=w200) -> ("States Out"=w199:string)  [unwired: 14 in]
          }
          frame "UI: Update FP Controls" {
            # "Do not put any code in this frame.\n(It is a separator no-op. You can make a copy of this frame to create a new UI frame)"
            n69 = Unbundle By Name(w203) -> ("UI Cluster.Parameter"=w201:dbl, "UI Cluster.Parameter 2"=w202:string)
            n70 = local write "Parameter 2"(w202) -> ()
            n71 = local write "Parameter"(w201) -> ()
            n72 = call <vilib>:"Add State(s) to Queue__jki_lib_state_machine.vi"("State(s) in (\"\")"=w207) -> ("States Out"=w206:string)  [unwired: 14 in]
          }
          frame "UI: Update FP Indicators" {
            # "do this way to have nicer UI or only display what you want"
            n73 = Unbundle By Name(w208) -> ("getAll"=w210:T5)
            n74 = Unbundle By Name(w210) -> ("Levy 1"=→"Levy 1":dbl, "Logger SMO"=→"Logger SMO":dbl, "SMO Boolean"=→"SMO Boolean":bool, "SMO String"=→"SMO string":string)
            n75 = call <vilib>:"Add State(s) to Queue__jki_lib_state_machine.vi"("State(s) in (\"\")"=w217) -> ("States Out"=w216:string)  [unwired: 14 in]
          }
          frame "UI: Cursor Set" {
            # "Argument"
            # "Initialize the User Interface, here.\n(this is called automatically, by the Macro: Init)"
            n76 = disable-structure shown="Default" {
              disable-tunnel: w220 -> [w225 w228]
              disable-tunnel: [w225 w227] -> w219
              disable-tunnel: w218 -> [_ w226]
              frame condition #0 {
              }
              frame condition #1 (active) {
                n77 = case shown="\"Busy\"" w226 {
                  tunnel: w228 -> [w230 w232]
                  tunnel: [w229 w231] -> w227
                  frame "Idle", Default {
                    n78 = call <vilib>:"Unset Busy.vi"("error in (no error)"=w230) -> ("error out"=w229:errorcluster)  [unwired: 10 in]
                  }
                  frame "Busy" {
                    n79 = call <vilib>:"Set Busy.vi"("error in (no error)"=w232) -> ("error out"=w231:errorcluster)  [unwired: 9 in, 1 out]
                  }
                }
              }
            }
            n80 = call <vilib>:"Add State(s) to Queue__jki_lib_state_machine.vi"("State(s) in (\"\")"=w224) -> ("States Out"=w223:string)  [unwired: 14 in]
          }
          frame "UI: Front Panel State" {
            # "Argument"
            # "Set Front Panel Open or Closed\n(Usage: \"UI: Front Panel State >> Open|Close\")"
            n81 = Unbundle By Name(w236) -> ("Core.Current VI Reference"=w235:refnum<vi>)
            n82 = disable-structure shown="Default" {
              disable-tunnel: w238 -> [w244 w267]
              disable-tunnel: [w243 w267] -> w237
              disable-tunnel: w235 -> [w242 _]
              disable-tunnel: w234 -> [w241 _]
              frame condition #0 (active) {
                n83 = case shown="\"Close\"" w241 {
                  tunnel: w244 -> [w248 w261]
                  tunnel: [w250 w262] -> w243
                  tunnel: w242 -> [w249 w259]
                  frame "Open", Default {
                    n84 = property class="VI"(reference=w249, error in=w248) -> (reference out=w246:refnum<vi>, error out=w247:errorcluster, "FP.State"=w245:T3)
                    n85 = case shown="\"Closed\"" w245 {
                      tunnel: [w253 w256] -> w250
                      tunnel: w247 -> [w252 w256]
                      tunnel: w246 -> [w251 _]
                      frame "Closed" {
                        n86 = invoke class="VI" method="FP.Open"(reference=w251, error in=w252, "Activate"=TRUE, "State"=T3."Standard") -> (error out=w253:errorcluster)  [unwired: 1 in, 4 out]
                      }
                      frame Default {
                      }
                    }
                  }
                  frame "Close" {
                    n87 = property class="VI"(reference=w259, error in=w261) -> (reference out=w258:refnum<vi>, error out=w260:errorcluster, "FP.State"=w257:T3)
                    n88 = case shown="Default" w257 {
                      tunnel: [w263 w266] -> w262
                      tunnel: w260 -> [w263 w265]
                      tunnel: w258 -> [_ w264]
                      frame "Invalid", "Closed" {
                      }
                      frame Default {
                        n89 = invoke class="VI" method="FP.Close"(reference=w264, error in=w265) -> (error out=w266:errorcluster)  [unwired: 1 in, 2 out]
                      }
                    }
                  }
                }
              }
              frame condition #1 {
              }
            }
            n90 = call <vilib>:"Add State(s) to Queue__jki_lib_state_machine.vi"("State(s) in (\"\")"=w240) -> ("States Out"=w239:string)  [unwired: 14 in]
          }
          frame "---------- Macro ----------" {
            # "Do not put any code in this frame.\n(It is a separator no-op. You can make a copy of this frame to create a new Macro frame)"
            n91 = call <vilib>:"Add State(s) to Queue__jki_lib_state_machine.vi"("State(s) in (\"\")"=w272) -> ("States Out"=w271:string)  [unwired: 14 in]
          }
          frame "Macro: Initialize" {
            w275 = "UI: Initialize\nMacro: Read UI Config\n//UI: Front Panel State >> Open"  # UI: Initialize Macro: Read UI Config //UI: Front Panel State >> Open
            # "Initialization Macro\n(This is called once, when the VI starts)"
            n92 = call <vilib>:"Add State(s) to Queue__jki_lib_state_machine.vi"("State(s) in Front (\"\")"="Data: Initialize\nInitialize Core Data\nEvents: Register", "State(s) in (\"\")"="Process: Sync", "State(s) at Back (\"\")"=w275) -> ("States Out"=w274:string)  [unwired: 12 in]
            n93 = call <vilib>:"Add State(s) to Queue__jki_lib_state_machine.vi"("State(s) in Front (\"\")"=w274, "State(s) in (\"\")"=w281) -> ("States Out"=w280:string)  [unwired: 13 in]
          }
          frame "Macro: Read UI Config" {
            # "Do not put any code in this frame.\n(It is a separator no-op. You can make a copy of this frame to create a new Macro frame)"
            n94 = call <vilib>:"Add State(s) to Queue__jki_lib_state_machine.vi"("State(s) in Front (\"\")"="Configuration: Initialize\nConfiguration: Read UI Config File\nUI: Update FP Controls" ("State(s) in Front (\"\")"), "State(s) in (\"\")"=w287) -> ("States Out"=w286:string)  [unwired: 13 in]
          }
          frame "Macro: Write UI Config" {
            # "Do not put any code in this frame.\n(It is a separator no-op. You can make a copy of this frame to create a new Macro frame)"
            n95 = call <vilib>:"Add State(s) to Queue__jki_lib_state_machine.vi"("State(s) in Front (\"\")"="Data: Set UI Cluster\nConfiguration: Write UI Config File" ("State(s) in Front (\"\")"), "State(s) in (\"\")"=w293) -> ("States Out"=w292:string)  [unwired: 13 in]
          }
          frame "Macro: Exit" {
            # "Exit Macro\n(This is called once, when the VI exits)"
            n96 = Unbundle By Name(w295) -> ("Core.Close Panel on Exit?"=w305:bool)
            n97 = Select(t="UI: Front Panel State >> Close", s=w305, f="") -> (s? t:f=w302:string)
            n98 = call <vilib>:"Add State(s) to Queue__jki_lib_state_machine.vi"("State(s) in Front (\"\")"="Data: Cleanup\nEvents: Unregister\nProcess: Self Terminate", "State(s) in (\"\")"="Process: Sync", "State(s) at Back (\"\")"="Exit") -> ("States Out"=w297:string)  [unwired: 12 in]
            n99 = call <vilib>:"Add State(s) to Queue__jki_lib_state_machine.vi"("State(s) in Front (\"\")"="Macro: Write UI Config", "State(s) in (\"\")"=w302, "State(s) at Back (\"\")"=w297) -> ("States Out"=w301:string)  [unwired: 12 in]
            n100 = call <vilib>:"Add State(s) to Queue__jki_lib_state_machine.vi"("State(s) in Front (\"\")"=w301, "State(s) in (\"\")"=w308) -> ("States Out"=w307:string)  [unwired: 13 in]
          }
          frame "---------- Process ----------" {
            # "Template Separator\n(You can make a copy of, or modify, this frame)"
            n101 = call <vilib>:"Add State(s) to Queue__jki_lib_state_machine.vi"("State(s) in (\"\")"=w313) -> ("States Out"=w312:string)  [unwired: 14 in]
          }
          frame "Process: Sync" {
            n102 = Unbundle By Name(w321) -> ("Instrument UI"=w317:refnum<class "Instrument UI.Template.lvclass">)
            n103 = call <vilib>:"WaitOnProcessSync.vi"("error in (no error)"=w316, "SMO"=w317) -> ("error out"=w315:errorcluster, "Don't run?"=w320:bool)  [unwired: 7 in, 1 out]
            n104 = Select(t="Data: Cleanup\nEvents: Unregister\nExit", s=w320, f="") -> (s? t:f=w314:string)
            n105 = call <vilib>:"Add State(s) to Queue__jki_lib_state_machine.vi"("State(s) in Front (\"\")"=w314, "State(s) in (\"\")"=w324) -> ("States Out"=w323:string)  [unwired: 13 in]
          }
          frame "Process: Self Terminate" {
            n106 = Unbundle By Name(w326) -> ("Instrument UI"=w325:refnum<class "Instrument UI.Template.lvclass">)
            n107 = call <vilib>:"SelfTerminate.vi"("error in (no error)"=w328, "SMO in"=w325) -> ("error out"=w327:errorcluster)  [unwired: 8 in, 1 out]
            n108 = call <vilib>:"Add State(s) to Queue__jki_lib_state_machine.vi"("State(s) in (\"\")"=w331) -> ("States Out"=w330:string)  [unwired: 14 in]
          }
          frame "---------- Events ----------" {
            # "Template Separator\n(You can make a copy of, or modify, this frame)"
            n109 = call <vilib>:"Add State(s) to Queue__jki_lib_state_machine.vi"("State(s) in (\"\")"=w336) -> ("States Out"=w335:string)  [unwired: 14 in]
          }
          frame "Events: Register" {
            # "Expand to add\nmore events"
            # "Base Class Protected Events"
            n110 = Unbundle By Name(w347) -> ("Instrument UI"=w338:refnum<class "Instrument UI.Template.lvclass">, "Instrument"=w337:refnum<class "Instrument.Template.lvclass">)
            n111 = call <vilib>:"GetProtectedEvents.vi"("SMO"=w338) -> ("error out"=w341:errorcluster, "SMO Protected Events"=w345:T9)  [unwired: 8 in, 1 out]
            n112 = call "Instrument.GetPublicEvents.vi"("Instrument"=w337) -> ("error out"=w339:errorcluster, "Instrument Public Events"=w340:T10)  [unwired: 8 in, 1 out]
            n113 = register-events(w345, w340) -> (reference out=w346:refnum<event-registration>, error out=w343:errorcluster)  [unwired: 2 in]
            n114 = Merge Errors(w339, w344, w343, w341) -> (w342:errorcluster)
            n115 = call <vilib>:"Add State(s) to Queue__jki_lib_state_machine.vi"("State(s) in (\"\")"=w349) -> ("States Out"=w348:string)  [unwired: 14 in]
          }
          frame "Events: Unregister" {
            n116 = Unregister For Events(event registration refnum=w352, error in=w351) -> (error out=w350:errorcluster)
            n117 = call <vilib>:"Add State(s) to Queue__jki_lib_state_machine.vi"("State(s) in (\"\")"=w355) -> ("States Out"=w354:string)  [unwired: 14 in]
          }
          frame "---------- Configuration ----------" {
            # "Do not put any code in this frame.\n(It is a separator no-op. You can make a copy of this frame to create a new UI frame)"
            n118 = call <vilib>:"Add State(s) to Queue__jki_lib_state_machine.vi"("State(s) in (\"\")"=w360) -> ("States Out"=w359:string)  [unwired: 14 in]
          }
          frame "Configuration: Initialize" {
            # "Do not put any code in this frame.\n(It is a separator no-op. You can make a copy of this frame to create a new UI frame)"
            n119 = Unbundle By Name(w363) -> ("Configuration"=w361:refnum<class "Configuration.lvclass">, "Instrument"=w362:refnum<class "Instrument.Template.lvclass">)
            n120 = call <vilib>:"GetName.vi"("error in (no error)"=w365, "SMO"=w362) -> ("error out"=w364:errorcluster, "Name"=w366:string)  [unwired: 6 in, 2 out]
            n121 = call "Default Path.vi"("error in (no error)"=w364, "Folder Name"=w366, "Configuration in"=w361) -> ("error out"=w367:errorcluster, "Configuration out"=w368:refnum<class "Configuration.lvclass">)  [unwired: 7 in]
            n122 = Bundle By Name(cluster=w363, "Configuration"=w368) -> (w369:T7)
            n123 = call <vilib>:"Add State(s) to Queue__jki_lib_state_machine.vi"("State(s) in (\"\")"=w372) -> ("States Out"=w371:string)  [unwired: 14 in]
          }
          frame "Configuration: Write UI Config File" {
            # "Do not put any code in this frame.\n(It is a separator no-op. You can make a copy of this frame to create a new Data frame)"
            n124 = Unbundle By Name(w377) -> ("Configuration"=w374:refnum<class "Configuration.lvclass">, "UI Cluster"=w376:T6)
            n125 = call "Write Configuration.vi"("error in (no error)"=w373, "Variant"=w376, "Configuration in"=w374) -> ("error out"=w375:errorcluster)  [unwired: 7 in, 1 out]
            n126 = call <vilib>:"Add State(s) to Queue__jki_lib_state_machine.vi"("State(s) in (\"\")"=w380) -> ("States Out"=w379:string)  [unwired: 14 in]
          }
          frame "Configuration: Read UI Config File" {
            # "Do not put any code in this frame.\n(It is a separator no-op. You can make a copy of this frame to create a new UI frame)"
            n127 = Unbundle By Name(w383) -> ("UI Cluster"=w386:T6, "Configuration"=w389:refnum<class "Configuration.lvclass">)
            n128 = call "Read Configuration.vi"("INI Fomatted Cluster Type"=w386, "error in (no error)"=w385, "Configuration in"=w389) -> ("error out"=w388:errorcluster, "Configuration"=w387:variant)  [unwired: 6 in, 1 out]
            n129 = Variant To Data(error in=w388, type=w386, Variant=w387) -> (data=w382:T6, error out=w384:errorcluster)
            n130 = Bundle By Name(cluster=w383, "UI Cluster"=w382) -> (w381:T7)
            n131 = call <vilib>:"Add State(s) to Queue__jki_lib_state_machine.vi"("State(s) in (\"\")"=w392) -> ("States Out"=w391:string)  [unwired: 14 in]
          }
          frame "---------- Action ----------" {
            n132 = Unbundle By Name(w395) -> ("Instrument UI"=w393:refnum<class "Instrument UI.Template.lvclass">)
            n133 = Bundle By Name(cluster=w395, "Instrument UI"=w393) -> (w394:T7)
            n134 = call <vilib>:"Add State(s) to Queue__jki_lib_state_machine.vi"("State(s) in (\"\")"=w399) -> ("States Out"=w398:string)  [unwired: 14 in]
          }
          frame "Action: Notify UI Closed" {
            # "Notify that the UI has been closed"
            n135 = Unbundle By Name(w400) -> ("Instrument UI"=w403:refnum<class "Instrument UI.Template.lvclass">)
            n136 = call <vilib>:"Hide.vi"("error in (no error)"=w402, "SMO.UI"=w403) -> ("error out"=w401:errorcluster)  [unwired: 8 in, 1 out]
            n137 = call <vilib>:"Add State(s) to Queue__jki_lib_state_machine.vi"("State(s) in (\"\")"=w406) -> ("States Out"=w405:string)  [unwired: 14 in]
          }
          frame "Action: getAll" {
            n138 = Unbundle By Name(w410) -> ("getAll"=w408:T5, "Instrument"=w413:refnum<class "Instrument.Template.lvclass">)
            n139 = call "GET ALL.vim"("type"=w408, "error in (no error)"=w411, "Instrument in"=w413) -> ("error out"=w415:errorcluster, "getAll"=w407:T5, "Instrument out"=w409:refnum<class "Instrument.Template.lvclass">)  [unwired: 6 in]
            n140 = Bundle By Name(cluster=w410, "Instrument"=w409, "getAll"=w407) -> (w412:T7)
            n141 = call <vilib>:"Add State(s) to Queue__jki_lib_state_machine.vi"("State(s) in Front (\"\")"="" ("State(s) in Front (\"\")"), "State(s) in (\"\")"=w418) -> ("States Out"=w417:string)  [unwired: 13 in]
          }
          frame "Action: setConfiguration" {
            n142 = Unbundle By Name(w421) -> ("Instrument"=w424:refnum<class "Instrument.Template.lvclass">, "Config Cluster"=w419:T4)
            n143 = call "SET CONFIG.vim"("error in (no error)"=w422, "Configuration"=w419, "Instrument in"=w424) -> ("error out"=w426:errorcluster, "Instrument out"=w420:refnum<class "Instrument.Template.lvclass">)  [unwired: 7 in]
            n144 = Bundle By Name(cluster=w421, "Instrument"=w420) -> (w423:T7)
            n145 = call <vilib>:"Add State(s) to Queue__jki_lib_state_machine.vi"("State(s) in Front (\"\")"="" ("State(s) in Front (\"\")"), "State(s) in (\"\")"=w429) -> ("States Out"=w428:string)  [unwired: 13 in]
          }
        }
      }
    }
    frame Error {
    }
  }
  n146 = call-parent "Process.vi"("error in"=w8, "Instrument UI in"=w7) -> ("error out"=w5:errorcluster, "Instrument UI out"=→"Example Instrument UI out":refnum<class "Instrument UI.Template.lvclass">)  [unwired: 8 in]
  n147 = Merge Errors(w5, w4) -> (→"error out":errorcluster)
